vi "Init.vi"(5 "Period (ms) in":i64, 6 "Players number in":u8=4, 7 "Player ID in":i64=1, 10 "Score to win in":u8=3, 11 "Game Board in":refnum<class "Game Board.lvclass">) -> (3 "Game Board out":refnum<class "Game Board.lvclass">)   [LabVIEW 2021, in "Game Board.lvclass"]
doc: "MIT Licence\nCopyright (c) 2024 David Grollier"
uses:
  Game Board.lvclass
  <vilib>/Utility/miscctls.llb/LVBoundsTypeDef.ctl
  Game Board.lvclass/Game Board.ctl
  <vilib>/Utility/miscctls.llb/LVPositionTypeDef.ctl
  Game Board Component/Fixed/Board/Rectangle/Rectangle.lvclass
  C:/Users/David/Documents/GameSoccerSpace/Source/Game Componants/Game Board Component/Fixed/Board/Board.lvclass
  Game Board Component/Fixed/Board/Goal post/Goal Post.lvclass
  Game Board Component/Fixed/Board/Board.lvclass
  C:/Users/David/Documents/GameSoccerSpace/Source/Game Componants/Game Board Component/Game Board Component.lvclass
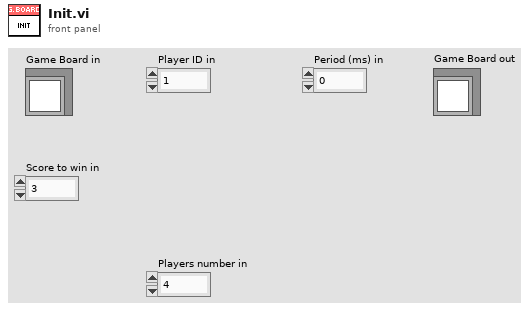
[diagram p1: front panel]
types:
  T1 = typedef "LVBoundsTypeDef.ctl" = cluster{"Width":u32, "Height":u32}
  T2 = cluster{"left":i16, "top":i16, "right":i16, "bottom":i16}[]
  T3 = typedef "LVPositionTypeDef.ctl" = cluster{"Left":i32, "Top":i32}
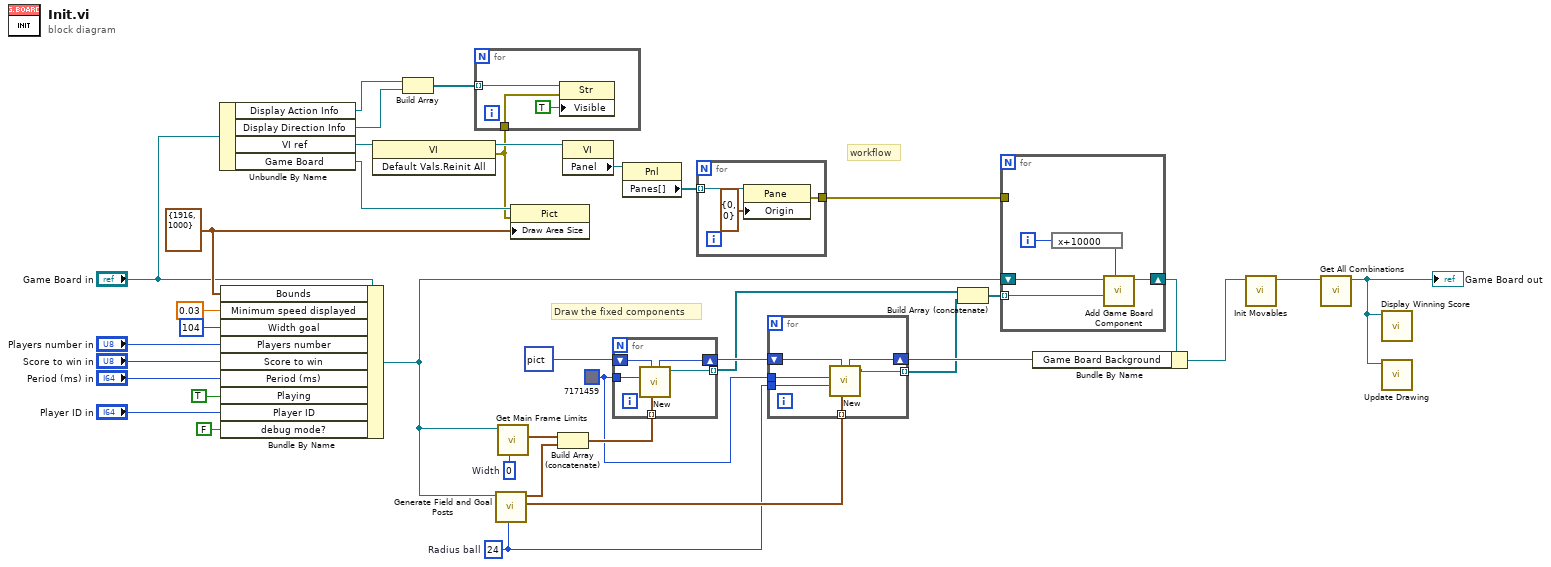
[diagram p0: block diagram]
diagram:
  w11 = T1 {"Width"=1916, "Height"=1000} ("Bounds in")
  w28 = u32 0  # Width
  w24 = u32 7171459 ("color in")
  w26 = i16 24  # Radius ball
  # "Draw the fixed components"
  # "workflow"
  n1 = Unbundle By Name("Game Board in") -> ("Display Action Info"=w4:refnum<vi>, "Display Direction Info"=w5:refnum<vi>, "VI ref"=w9:refnum<vi>, "Game Board"=w16:refnum<vi>)
  n2 = Bundle By Name(cluster="Game Board in", "Bounds"=w11, "Minimum speed displayed"=0.03, "Width goal"=u32 104, "Players number"="Players number in", "Score to win"="Score to win in", "Period (ms)"="Period (ms) in", "Playing"=TRUE, "Player ID"="Player ID in", "debug mode?"=FALSE) -> (w17:refnum<class "Game Board.lvclass">)
  n3 = invoke class="VI" method="Default Vals.Reinit All"(reference=w9) -> (reference out=w8:refnum<vi>, error out=w6:errorcluster)  [unwired: 2 in, 1 out]
  n4 = Build Array(w4, w5) -> (w3:refnum<vi>[])
  n5 = for {
    tunnel: w6 -> [w41]
    tunnel: w3 -> [w39] mode=indexing
    n6 = property class="Str"(reference=w39, error in=w41, "Visible"=TRUE) -> ()  [unwired: 2 out]
  }
  n7 = call "Generate Field and Goal Posts.vi"("Height"=w26, "Game Board in"=w17) -> ("Goal post out"=w27:T2, "Field limit out"=w34:T2)  [unwired: 8 in]
  n8 = call "Get Main Frame Limits.vi"("Width"=w28, "Game Board in"=w17) -> ("rect out"=w29:T2)  [unwired: 9 in]
  n9 = property class="Pict"(reference=w16, error in=w6, "Draw Area Size"=w11) -> ()  [unwired: 2 out]
  n10 = Build Array (concatenate)(w29, w34) -> (w33:T2)
  n11 = property class="VI"(reference=w8) -> ("Panel"=w15:refnum<vi>)  [unwired: 1 in, 2 out]
  n12 = for {
    tunnel: w33 -> [w46] mode=indexing
    tunnel: w24 -> [w45]
    shift-right: [w43] -> w36
    shift-left: picture data[5B] ("Game Board Background") -> [w44]
    tunnel: [w42] -> w31 mode=indexing
    n13 = call "New.vi"("rect in"=w46, "picture in"=w44, "color in"=w45) -> ("Rectangle out"=w42:refnum<class "Rectangle.lvclass">, "picture out"=w43:picture)  [unwired: 7 in]
  }
  n14 = property class="Pnl"(reference=w15) -> ("Panes[]"=w22:refnum<vi>[])  [unwired: 1 in, 2 out]
  n15 = for {
    tunnel: w22 -> [w48] mode=indexing
    tunnel: [w47] -> w7
    n16 = property class="Pane"(reference=w48, "Origin"=T3 {"Left"=0, "Top"=0} ("Position")) -> (error out=w47:errorcluster)  [unwired: 1 in, 1 out]
  }
  n17 = for {
    tunnel: w27 -> [w55] mode=indexing
    tunnel: w24 -> [w54]
    tunnel: w26 -> [w53]
    shift-right: [w51] -> w38
    shift-left: w36 -> [w52]
    tunnel: [w50] -> w32 mode=indexing
    n18 = call "New.vi"("rect in"=w55, "picture"=w52, "Radius in"=w53, "color in"=w54) -> ("Goal post out"=w50:refnum<class "Goal Post.lvclass">, "picture out"=w51:picture)  [unwired: 6 in]
  }
  n19 = Build Array (concatenate)(w31, w32) -> (w30:refnum<class "Board.lvclass">[])
  n20 = for {
    tunnel: w30 -> [w58] mode=indexing
    shift-right: [w56] -> w35
    shift-left: w17 -> [w57]
    tunnel: w7 -> [_]
    i -> [w60]
    n21 = expression code="x+10000"(w60) -> (w59:i32)
    n22 = call "Add Game Board Component.vi"("Game Board Component in"=w58, "Index in"=w59, "Game Board in"=w57) -> ("Game Board out"=w56:refnum<class "Game Board.lvclass">)  [unwired: 8 in]
  }
  n23 = Bundle By Name(cluster=w35, "Game Board Background"=w38) -> (w21:refnum<class "Game Board.lvclass">)
  n24 = call "Init Movables.vi"("Game Board in"=w21) -> ("Game Board out"=w20:refnum<class "Game Board.lvclass">)  [unwired: 10 in]
  n25 = call "Get All Combinations.vi"("Game Board in"=w20) -> ("Game Board out"=w19:refnum<class "Game Board.lvclass">)  [unwired: 10 in]
  "Game Board out" <- w19
  n26 = call "Display Winning Score.vi"("Game Board in"=w19) -> ()  [unwired: 11 in]
  n27 = call "Update Drawing.vi"("Game Board in"=w19) -> ()  [unwired: 11 in]
